vi "VerifErrors.vi"(8 "error in (no error)":errorcluster, 11 "S4GUI in":refnum<class "S4GUI.lvclass">) -> (0 "error out":errorcluster, 2 "Error value":u32, 3 "S4GUI out":refnum<class "S4GUI.lvclass">)   [LabVIEW 2018, in "S4GUI.lvclass"]
uses:
  S4GUI.lvclass
  S4GUI.lvclass/S4GUI.ctl
  Acquisition/Acquisition.lvclass
  Channel/Channel.lvclass
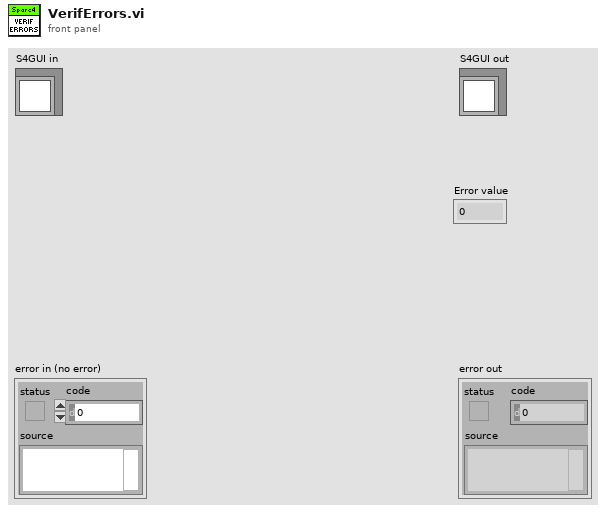
[diagram p1: front panel]
types:
  T1 = cluster{"Texp":dbl, "Nimages":u32, "InitialLine":u32, "FinalLine":u32, "InitialColumn":u32, "FinalColumn":u32, "EmGain":u32, "Cooler Off":bool, "CyclesDone":u32, "SequesDone":u32, "UsedDiskSpace":u16, "Error":bool}
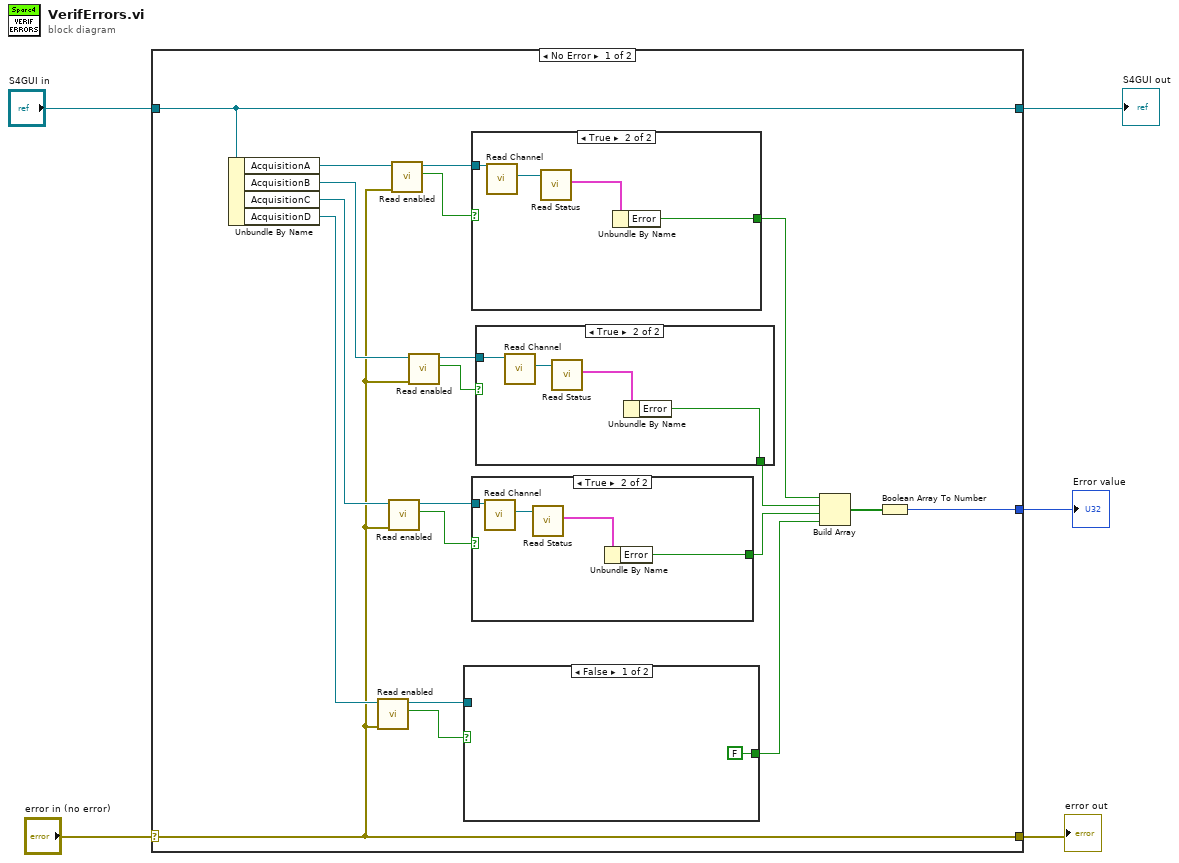
[diagram p0: block diagram]
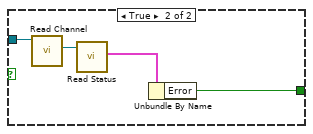
[diagram p2: hidden frame]
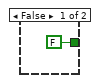
[diagram p3: hidden frame]
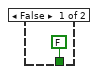
[diagram p4: hidden frame]
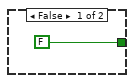
[diagram p5: hidden frame]
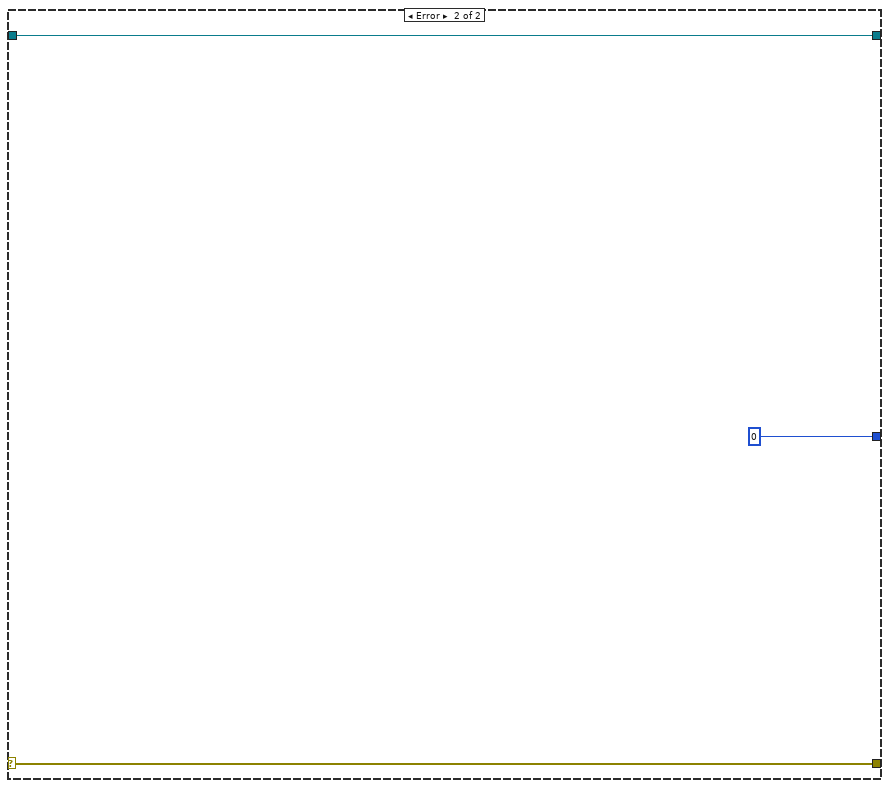
[diagram p6: hidden frame]
diagram:
  n1 = case shown="No Error" "error in (no error)" {
    selector: "error in (no error)" -> [w12 w48]
    tunnel: [w12 w48] -> w1
    tunnel: [w25 w47] -> w2
    tunnel: "S4GUI in" -> [w25 w47]
    tunnel: [w6 u32 0] -> w3
    frame No Error {
      n2 = Unbundle By Name(w25) -> ("AcquisitionA"=w24:refnum<class "Acquisition.lvclass">, "AcquisitionB"=w21:refnum<class "Acquisition.lvclass">, "AcquisitionC"=w18:refnum<class "Acquisition.lvclass">, "AcquisitionD"=w15:refnum<class "Acquisition.lvclass">)
      n3 = call-dynamic "Read enabled.vi"("error in (no error)"=w12, "Server in"=w15) -> ("enabled"=w13:bool, "Server out"=w14:refnum<class "Acquisition.lvclass">)  [unwired: 7 in, 1 out]
      n4 = call-dynamic "Read enabled.vi"("error in (no error)"=w12, "Server in"=w18) -> ("enabled"=w16:bool, "Server out"=w17:refnum<class "Acquisition.lvclass">)  [unwired: 7 in, 1 out]
      n5 = call-dynamic "Read enabled.vi"("error in (no error)"=w12, "Server in"=w24) -> ("enabled"=w22:bool, "Server out"=w23:refnum<class "Acquisition.lvclass">)  [unwired: 7 in, 1 out]
      n6 = call-dynamic "Read enabled.vi"("error in (no error)"=w12, "Server in"=w21) -> ("enabled"=w19:bool, "Server out"=w20:refnum<class "Acquisition.lvclass">)  [unwired: 7 in, 1 out]
      n7 = case shown="False" w13 {
        tunnel: w14 -> [_ w30]
        tunnel: [FALSE w27] -> w8
        frame False {
        }
        frame True {
          n8 = call-dynamic "Read Channel.vi"("Acquisition in"=w30) -> ("Channel.lvclass"=w28:refnum<class "Channel.lvclass">)  [unwired: 8 in, 2 out]
          n9 = call-dynamic "Read Status.vi"("Channel in"=w28) -> ("Status"=w29:T1)  [unwired: 8 in, 2 out]
          n10 = Unbundle By Name(w29) -> ("Error"=w27:bool)
        }
      }
      n11 = case shown="True" w22 {
        tunnel: [FALSE w42] -> w11
        tunnel: w23 -> [_ w45]
        frame False {
        }
        frame True {
          n12 = call-dynamic "Read Channel.vi"("Acquisition in"=w45) -> ("Channel.lvclass"=w44:refnum<class "Channel.lvclass">)  [unwired: 8 in, 2 out]
          n13 = call-dynamic "Read Status.vi"("Channel in"=w44) -> ("Status"=w43:T1)  [unwired: 8 in, 2 out]
          n14 = Unbundle By Name(w43) -> ("Error"=w42:bool)
        }
      }
      n15 = case shown="True" w16 {
        tunnel: w17 -> [_ w35]
        tunnel: [FALSE w32] -> w9
        frame False {
        }
        frame True {
          n16 = call-dynamic "Read Channel.vi"("Acquisition in"=w35) -> ("Channel.lvclass"=w33:refnum<class "Channel.lvclass">)  [unwired: 8 in, 2 out]
          n17 = call-dynamic "Read Status.vi"("Channel in"=w33) -> ("Status"=w34:T1)  [unwired: 8 in, 2 out]
          n18 = Unbundle By Name(w34) -> ("Error"=w32:bool)
        }
      }
      n19 = case shown="True" w19 {
        tunnel: w20 -> [_ w40]
        tunnel: [FALSE w37] -> w10
        frame False {
        }
        frame True {
          n20 = call-dynamic "Read Channel.vi"("Acquisition in"=w40) -> ("Channel.lvclass"=w38:refnum<class "Channel.lvclass">)  [unwired: 8 in, 2 out]
          n21 = call-dynamic "Read Status.vi"("Channel in"=w38) -> ("Status"=w39:T1)  [unwired: 8 in, 2 out]
          n22 = Unbundle By Name(w39) -> ("Error"=w37:bool)
        }
      }
      n23 = Build Array(w11, w10, w9, w8) -> (w7:bool[])
      n24 = Boolean Array To Number(Boolean array=w7) -> (number=w6:u32)
    }
    frame Error {
    }
  }
  "error out" <- w1
  "S4GUI out" <- w2
  "Error value" <- w3
